vi "TEST_Progress.vi"(8 "error in (no error)":errorcluster) -> (0 "error out":errorcluster)   [LabVIEW 2021]
uses:
  Progress.lvclass
panel:
  out "Horizontal Progress Bar":u64(slide) caption="Loop 20 of 20" scale=0.0..40.0
  out "Slide 3":u64(slide) scale=0.0..40.0
  out "Slide 2":dbl(slide) scale=0.0..20.0
  out "Slide":u64(slide) scale=0.0..20.0
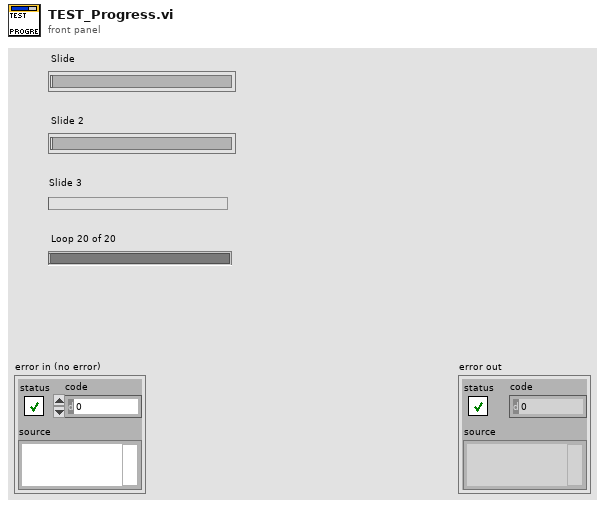
[diagram p1: front panel]
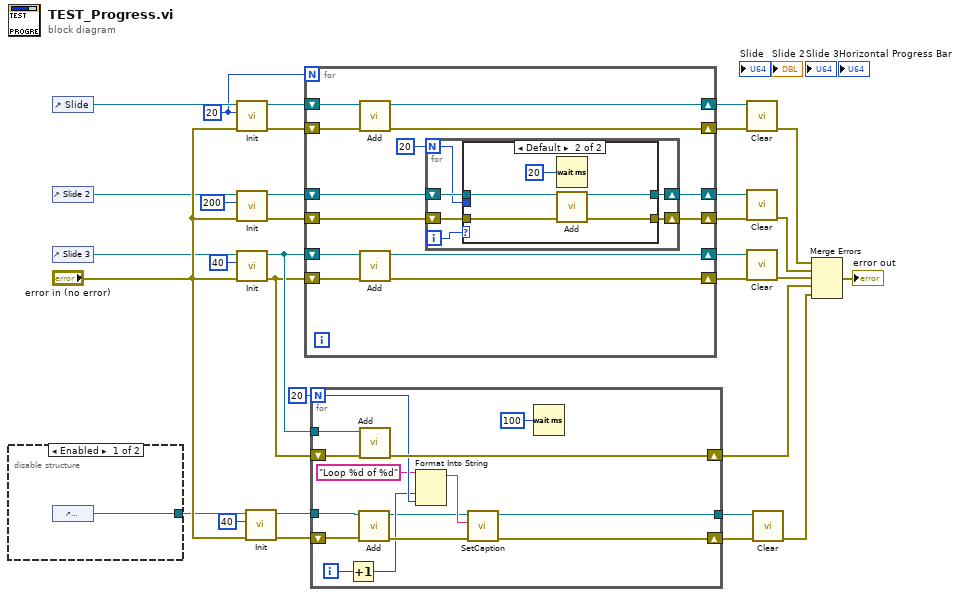
[diagram p0: block diagram]
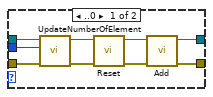
[diagram p3: hidden frame]
diagram:
  w10 = u64 20 ("Nb Element")
  n1 = disable-structure shown="Enabled" {
    disable-tunnel: [w33 _] -> w28
    frame Enabled {
      n2 = control-ref of="Horizontal Progress Bar"() -> (w33:refnum<vi>)
    }
    frame Disabled {
    }
  }
  n3 = control-ref of="Slide"() -> (w31:refnum<vi>)
  n4 = control-ref of="Slide 2"() -> (w30:refnum<vi>)
  n5 = control-ref of="Slide 3"() -> (w29:refnum<vi>)
  n6 = call "Init.vi"("error in (no error)"="error in (no error)", "Nb Element"=w10, "Slide Refnum"=w31) -> ("error out"=w26:errorcluster, "Progress out"=w27:refnum<class "Progress.lvclass">)  [unwired: 7 in]
  n7 = call "Init.vi"("error in (no error)"="error in (no error)", "Nb Element"=u64 200, "Slide Refnum"=w30) -> ("error out"=w21:errorcluster, "Progress out"=w22:refnum<class "Progress.lvclass">)  [unwired: 7 in]
  n8 = call "Init.vi"("error in (no error)"="error in (no error)", "Nb Element"=u64 40, "Slide Refnum"=w29) -> ("error out"=w12:errorcluster, "Progress out"=w13:refnum<class "Progress.lvclass">)  [unwired: 7 in]
  n9 = call "Init.vi"("error in (no error)"="error in (no error)", "Nb Element"=u64 40, "Slide Refnum"=w28) -> ("error out"=w5:errorcluster, "Progress out"=w6:refnum<class "Progress.lvclass">)  [unwired: 7 in]
  n10 = for {
    N: w10 -> [_]
    shift-right: [w44] -> w25
    shift-left: w27 -> [w45]
    shift-right: [w43] -> w24
    shift-left: w26 -> [w46]
    shift-right: [w36] -> w20
    shift-left: w22 -> [w42]
    shift-right: [w35] -> w19
    shift-left: w21 -> [w41]
    shift-right: [w38] -> w17
    shift-left: w13 -> [w37]
    shift-right: [w40] -> w18
    shift-left: w12 -> [w39]
    n11 = call "Add.vi"("error in (no error)"=w46, "Progress in"=w45) -> ("error out"=w43:errorcluster, "Progress out"=w44:refnum<class "Progress.lvclass">)  [unwired: 8 in]
    n12 = call "Add.vi"("error in (no error)"=w39, "Progress in"=w37) -> ("error out"=w40:errorcluster, "Progress out"=w38:refnum<class "Progress.lvclass">)  [unwired: 8 in]
    n13 = for {
      N: 20 -> [w47]
      shift-right: [w52] -> w36
      shift-left: w42 -> [w49]
      shift-right: [w51] -> w35
      shift-left: w41 -> [w48]
      i -> [w50]
      n14 = case shown="Default" w50 {
        tunnel: [w58 w66] -> w52
        tunnel: [w60 w65] -> w51
        tunnel: w49 -> [w55 w63]
        tunnel: w48 -> [w61 w62]
        tunnel: w47 -> [w53 _]
        frame ..0 {
          n15 = call "UpdateNumberOfElement.vi"("error in (no error)"=w61, "Nb Element"=w53, "Progress in"=w55) -> ("error out"=w56:errorcluster, "Progress out"=w54:refnum<class "Progress.lvclass">)  [unwired: 7 in]
          n16 = call "Reset.vi"("error in (no error)"=w56, "Progress in"=w54) -> ("error out"=w57:errorcluster, "Progress out"=w59:refnum<class "Progress.lvclass">)  [unwired: 8 in]
          n17 = call "Add.vi"("error in (no error)"=w57, "Progress in"=w59) -> ("error out"=w60:errorcluster, "Progress out"=w58:refnum<class "Progress.lvclass">)  [unwired: 8 in]
        }
        frame Default {
          n18 = Wait (ms)(milliseconds to wait=u32 20) -> ()  [unwired: 1 out]
          n19 = call "Add.vi"("error in (no error)"=w62, "Progress in"=w63) -> ("error out"=w65:errorcluster, "Progress out"=w66:refnum<class "Progress.lvclass">)  [unwired: 8 in]
        }
      }
    }
  }
  n20 = for {
    N: 20 -> [w73]
    tunnel: w13 -> [w81]
    shift-right: [w79] -> w11
    shift-left: w12 -> [w80]
    tunnel: w6 -> [w77]
    shift-right: [w74] -> w2
    shift-left: w5 -> [w76]
    tunnel: [w67] -> w4
    i -> [w72]
    n21 = Increment(x=w72) -> (x+1=w71:i32)
    n22 = call "Add.vi"("error in (no error)"=w76, "Progress in"=w77) -> ("error out"=w75:errorcluster, "Progress out"=w68:refnum<class "Progress.lvclass">)  [unwired: 8 in]
    n23 = call "Add.vi"("error in (no error)"=w80, "Progress in"=w81) -> ("error out"=w79:errorcluster)  [unwired: 8 in, 1 out]
    n24 = Format Into String(format string="Loop %d of %d", w71, w73) -> (resulting string=w69:string)  [unwired: 2 in, 1 out]
    n25 = call "SetCaption.vi"("error in (no error)"=w75, "Caption"=w69, "Progress in"=w68) -> ("error out"=w74:errorcluster, "Progress out"=w67:refnum<class "Progress.lvclass">)  [unwired: 7 in]
    n26 = Wait (ms)(milliseconds to wait=u32 100) -> ()  [unwired: 1 out]
  }
  n27 = call "Clear.vi"("error in (no error)"=w24, "Progress in"=w25) -> ("error out"=w16:errorcluster)  [unwired: 9 in]
  n28 = call "Clear.vi"("error in (no error)"=w19, "Progress in"=w20) -> ("error out"=w15:errorcluster)  [unwired: 9 in]
  n29 = call "Clear.vi"("error in (no error)"=w18, "Progress in"=w17) -> ("error out"=w14:errorcluster)  [unwired: 9 in]
  n30 = call "Clear.vi"("error in (no error)"=w2, "Progress in"=w4) -> ("error out"=w1:errorcluster)  [unwired: 9 in]
  n31 = Merge Errors(w16, w15, w14, w11, w1) -> (→"error out":errorcluster)
